vi "SM-SG Main.vi"() -> ()   [LabVIEW 2018]
doc: "Gerador de Sinal estruturado em formato de máquina de estados."
uses:
  Controls/Botao_Senoidal.ctl
  Controls/SM-SG State.ctl
  Controls/SM-SG Data.ctl
  <vilib>/DAQmx/write.llb/DAQmx Write (Analog Wfm 1Chan NSamp).vi
  <vilib>/Waveform/WDTOps.llb/WDT Append Waveforms DBL.vi
  <vilib>/DAQmx/create/channels.llb/DAQmx Create Channel (AO-Voltage-Basic).vi
  <vilib>/DAQmx/configure/timing.llb/DAQmx Timing (Sample Clock).vi
  <vilib>/DAQmx/miscellaneous.llb/DAQmx Fill In Error Info.vi
  <vilib>/measure/NI_MABase.lvlib
  <resource>/objmgr/daqmx.rc
panel:
  in  "% Descida":dbl(knob)=25.01013479174359 max=100.0 step=1.0 scale=0.0..100.0
  in  "% High":dbl(knob)=25.0 min=0.0 max=100.0 step=1.0 scale=0.0..100.0
  in  "% Subida":dbl(knob)=25.0 min=0.0 max=100.0 step=1.0 scale=0.0..100.0
  in  "physical channels 2":tag
  in  "Duty Cycle":dbl(knob) min=0.0 max=100.0 step=1.0 scale=0.0..100.0
  in  "Fase":dbl(knob) min=-180.0 max=180.0 step=5.0 scale=-180.0..180.0
  in  "Offset":dbl(slide) min=-5.5 max=5.5 step=0.1 scale=-5.5..5.5
  in  "Ciclos":i64(knob)=1 min=1 max=10 scale=1.0..10.0
  in  "Frequência":dbl=1.0 min=0.01 max=100000.0 step=0.001
  in  "Amplitude [Vp]":dbl(knob)=5.1000000000000005 caption="Amplitude" min=0.0 max=10.0 step=0.01 scale=0.0..10.0
  in  "Tipo de forma de onda":T2
  in  "Validar":bool
  in  "Parar":bool
  in  "Remove":bool
  out "Xf":dbl
  out "X0":dbl
  in  "Gerar":bool
  out "Sinal":waveform(dbl)(graph)={"t0"=timestamp(0 s since 1904-01-01), "dt"=0.0002, "Y"=[]}
  out "Onda":waveform(dbl)(graph)
  in  "Abrir":bool
  in  "Salvar":bool
  in  "Limpa":bool
  in  "Adicionar":bool
  in  "Stop Button":bool
  # "Onda Configurada"
  # "Configurações da Onda"
  # "Sinal Construído"
  # "Edição do Sinal Construído"
  # "Geração do Sinal"
  # "Cursores"
  # "Canal de Saída"
  # "X1"
  # "X2"
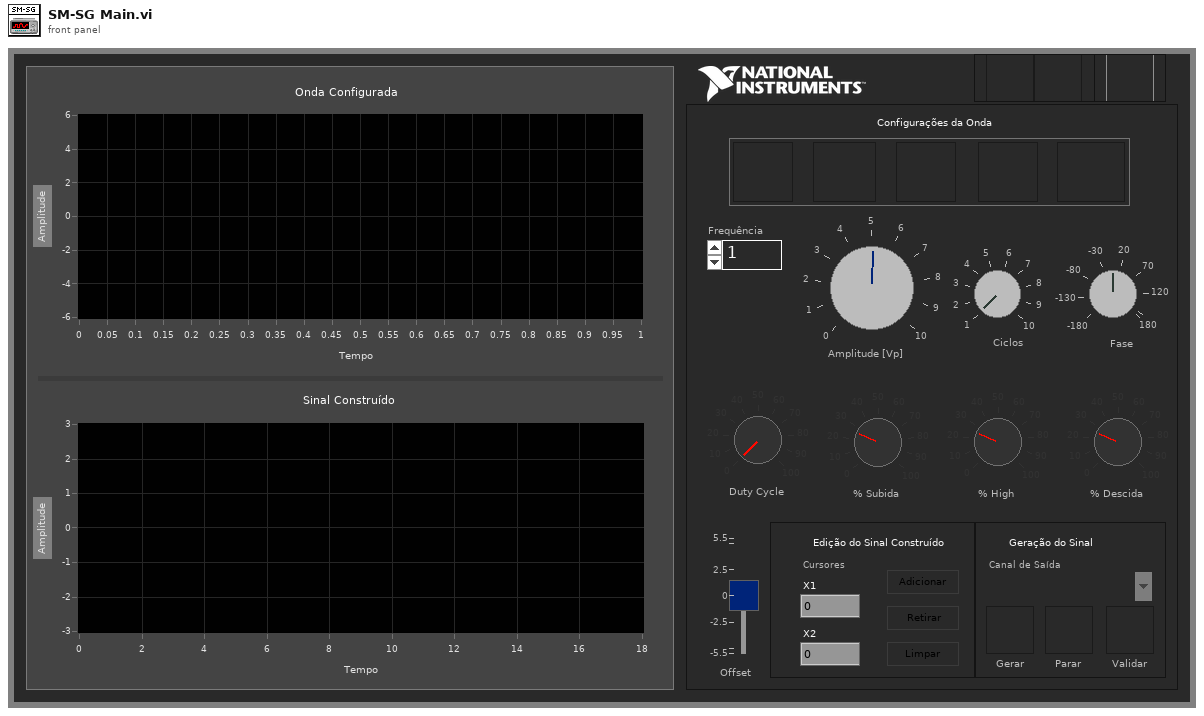
[diagram p1: front panel]
types:
  T1 = typedef "Botao_Senoidal.ctl" = bool
  T2 = cluster{"Sine Wave":T1, "Triangle Wave":bool, "Square Wave":bool, "Sawtooth":bool, "Trapezoidal":bool}
  T3 = typedef "SM-SG Data.ctl" = cluster{"Onda":waveform(dbl), "Sinal":waveform(dbl), "Parâmetros Onda Trapezoidal":cluster{"% Subida ":dbl, "% High ":dbl, "% Descida ":dbl}, "SinalGerado":waveform(dbl), "Analog Output":refnum<k21>, "Analog Input":refnum<k21>, "Tipo de forma de onda ":enum16{"Sine Wave", "Triangle Wave", "Square Wave", "Sawtooth Wave", "Trapezoidal Wave"}, "Amplitude ":dbl, "Frequencia ":dbl, "Ciclos ":dbl, "Fase ":dbl, "Offset":dbl, "Duty Cycle ":dbl}
  T4 = typedef "SM-SG State.ctl" = enum16{"Inicio", "Aguarda Evento", "Desenha Onda", "Mostra Onda", "Mostra Sinal", "Limpa Gráfico", "Adicionar", "Remover", "Salvar", "Carregar", "Gera onda", "Valida onda", "Parar geração", "Gerenciador Erro", "Sair"}
  T5 = enum16{"Sine Wave", "Triangle Wave", "Square Wave", "Sawtooth Wave", "Trapezoidal Wave"}
  T6 = enum16{"open", "open or create", "create or replace", "create", "open (read-only)"}
  T7 = enum16{"Sine Wave", "Triangle Wave", "Square Wave", "Sawtooth Wave", "Trapezoidal Wave"}[]
  T8 = cluster{"% Subida ":dbl, "% High ":dbl, "% Descida ":dbl}
  T9 = typedef "LVCursorListTypeDef.ctl" = cluster{"Name":string, "Color":u32, "Style":u8, "Point Style":u8, "Name Visible":bool, "Allow Drag":bool, "Cursor Mode":u32, "Plot":i32, "Index":i32, "Position":cluster{"X":dbl, "Y":dbl}, "X Scale":u32, "Y Scale":u32, "Watch Plots":i32[], "Watch All Plots":bool, "Plot Area":i32, "Label Offset":cluster{"X":dbl, "Y":dbl}}[]
  T10 = cluster{"CrsrList[0]":cluster{"Name":string, "Color":u32, "Style":u8, "Point Style":u8, "Name Visible":bool, "Allow Drag":bool, "Cursor Mode":u32, "Plot":i32, "Index":i32, "Position":cluster{"X":dbl, "Y":dbl}, "X Scale":u32, "Y Scale":u32, "Watch Plots":i32[], "Watch All Plots":bool, "Plot Area":i32, "Label Offset":cluster{"X":dbl, "Y":dbl}}, "CrsrList[1]":cluster{"Name":string, "Color":u32, "Style":u8, "Point Style":u8, "Name Visible":bool, "Allow Drag":bool, "Cursor Mode":u32, "Plot":i32, "Index":i32, "Position":cluster{"X":dbl, "Y":dbl}, "X Scale":u32, "Y Scale":u32, "Watch Plots":i32[], "Watch All Plots":bool, "Plot Area":i32, "Label Offset":cluster{"X":dbl, "Y":dbl}}, "CrsrList[2]":cluster{"Name":string, "Color":u32, "Style":u8, "Point Style":u8, "Name Visible":bool, "Allow Drag":bool, "Cursor Mode":u32, "Plot":i32, "Index":i32, "Position":cluster{"X":dbl, "Y":dbl}, "X Scale":u32, "Y Scale":u32, "Watch Plots":i32[], "Watch All Plots":bool, "Plot Area":i32, "Label Offset":cluster{"X":dbl, "Y":dbl}}, "CrsrList[3]":cluster{"Name":string, "Color":u32, "Style":u8, "Point Style":u8, "Name Visible":bool, "Allow Drag":bool, "Cursor Mode":u32, "Plot":i32, "Index":i32, "Position":cluster{"X":dbl, "Y":dbl}, "X Scale":u32, "Y Scale":u32, "Watch Plots":i32[], "Watch All Plots":bool, "Plot Area":i32, "Label Offset":cluster{"X":dbl, "Y":dbl}}, "CrsrList[4]":cluster{"Name":string, "Color":u32, "Style":u8, "Point Style":u8, "Name Visible":bool, "Allow Drag":bool, "Cursor Mode":u32, "Plot":i32, "Index":i32, "Position":cluster{"X":dbl, "Y":dbl}, "X Scale":u32, "Y Scale":u32, "Watch Plots":i32[], "Watch All Plots":bool, "Plot Area":i32, "Label Offset":cluster{"X":dbl, "Y":dbl}}, "CrsrList[5]":cluster{"Name":string, "Color":u32, "Style":u8, "Point Style":u8, "Name Visible":bool, "Allow Drag":bool, "Cursor Mode":u32, "Plot":i32, "Index":i32, "Position":cluster{"X":dbl, "Y":dbl}, "X Scale":u32, "Y Scale":u32, "Watch Plots":i32[], "Watch All Plots":bool, "Plot Area":i32, "Label Offset":cluster{"X":dbl, "Y":dbl}}, "CrsrList[6]":cluster{"Name":string, "Color":u32, "Style":u8, "Point Style":u8, "Name Visible":bool, "Allow Drag":bool, "Cursor Mode":u32, "Plot":i32, "Index":i32, "Position":cluster{"X":dbl, "Y":dbl}, "X Scale":u32, "Y Scale":u32, "Watch Plots":i32[], "Watch All Plots":bool, "Plot Area":i32, "Label Offset":cluster{"X":dbl, "Y":dbl}}, "CrsrList[7]":cluster{"Name":string, "Color":u32, "Style":u8, "Point Style":u8, "Name Visible":bool, "Allow Drag":bool, "Cursor Mode":u32, "Plot":i32, "Index":i32, "Position":cluster{"X":dbl, "Y":dbl}, "X Scale":u32, "Y Scale":u32, "Watch Plots":i32[], "Watch All Plots":bool, "Plot Area":i32, "Label Offset":cluster{"X":dbl, "Y":dbl}}, "CrsrList[8]":cluster{"Name":string, "Color":u32, "Style":u8, "Point Style":u8, "Name Visible":bool, "Allow Drag":bool, "Cursor Mode":u32, "Plot":i32, "Index":i32, "Position":cluster{"X":dbl, "Y":dbl}, "X Scale":u32, "Y Scale":u32, "Watch Plots":i32[], "Watch All Plots":bool, "Plot Area":i32, "Label Offset":cluster{"X":dbl, "Y":dbl}}}
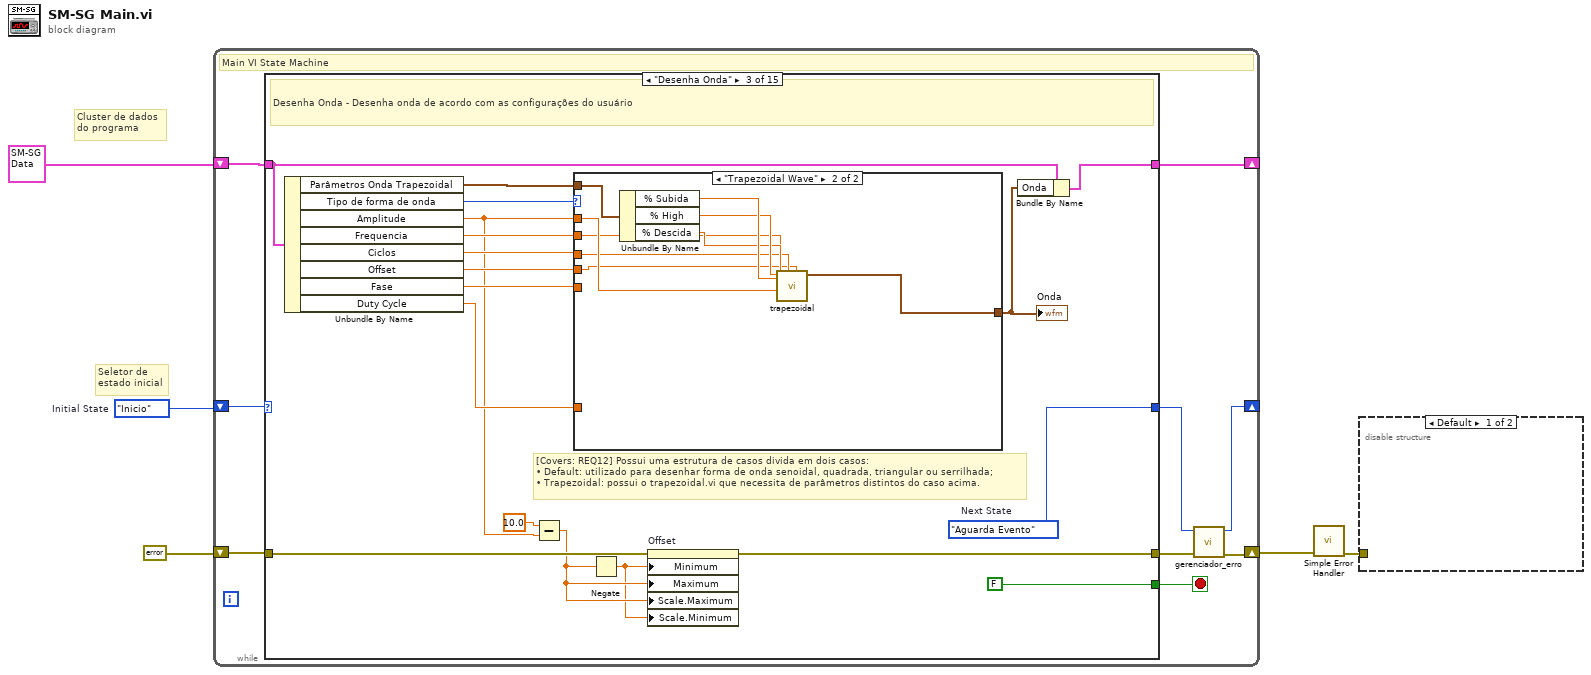
[diagram p0: block diagram]
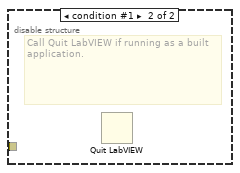
[diagram p2: hidden frame]
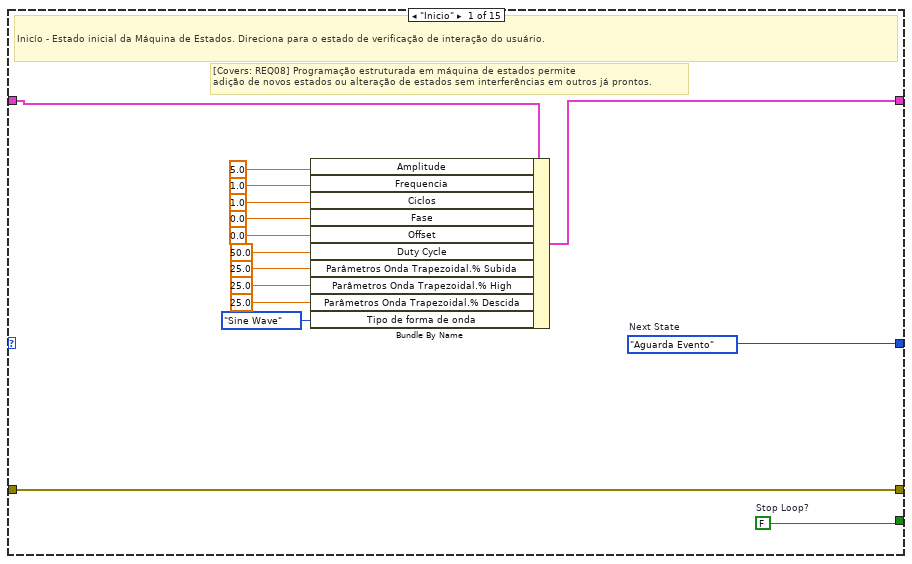
[diagram p3: hidden frame]
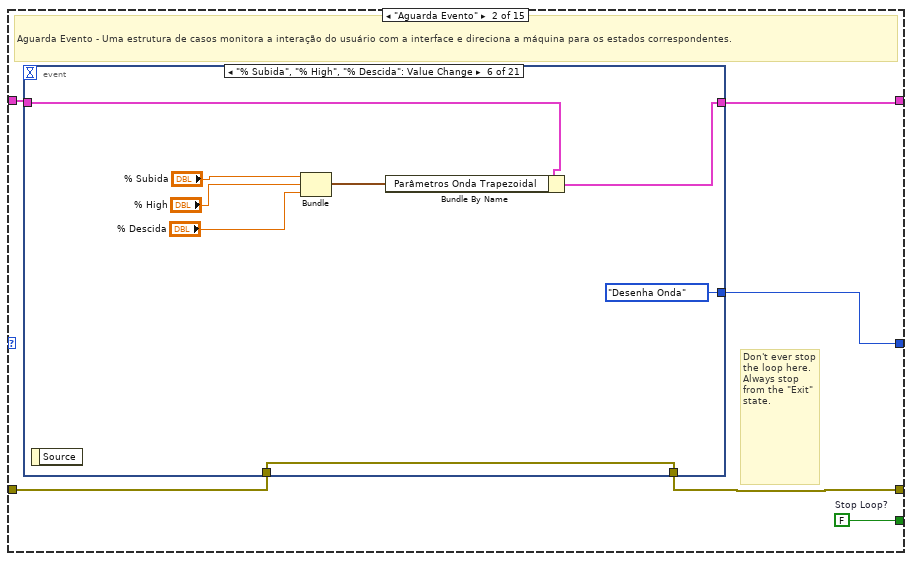
[diagram p4: hidden frame]
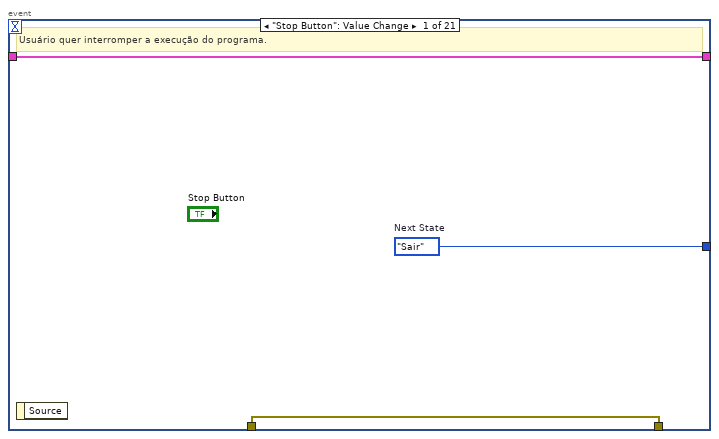
[diagram p5: hidden frame]
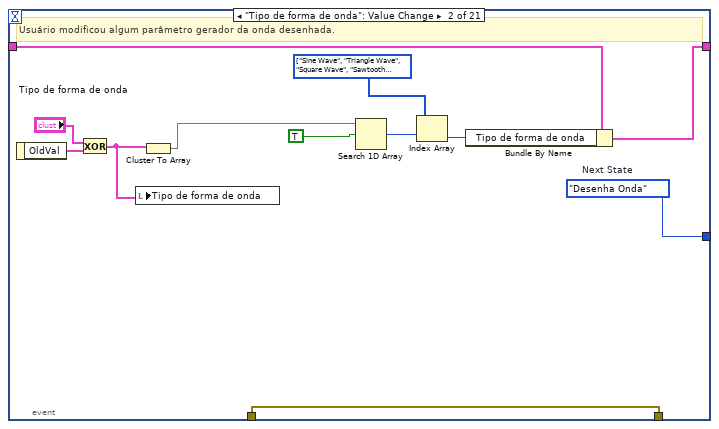
[diagram p6: hidden frame]
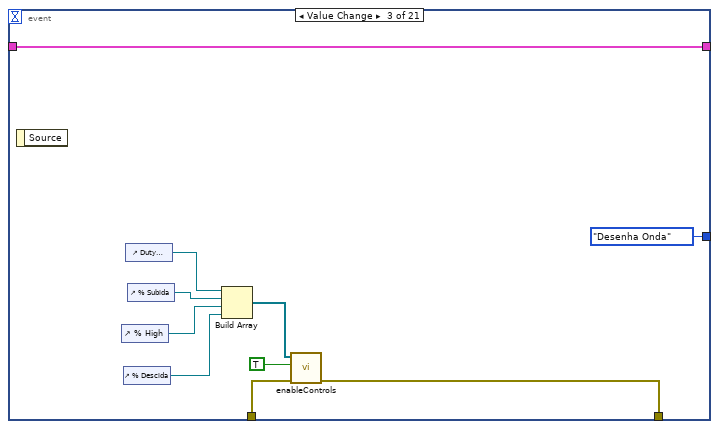
[diagram p7: hidden frame]
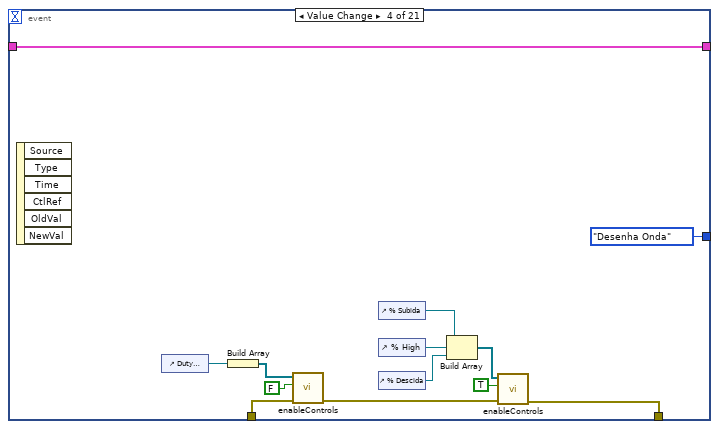
[diagram p8: hidden frame]
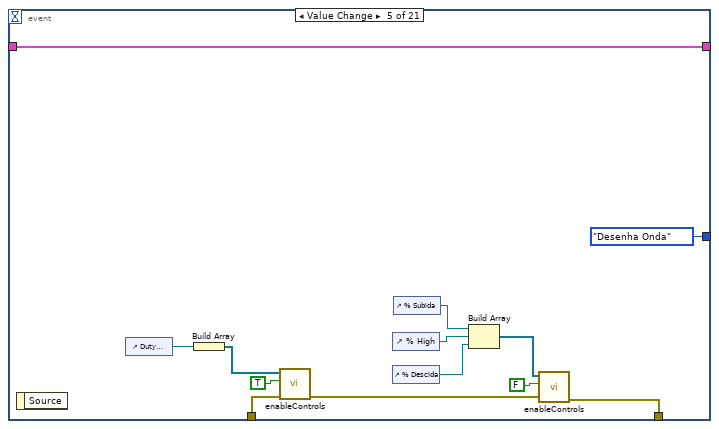
[diagram p9: hidden frame]
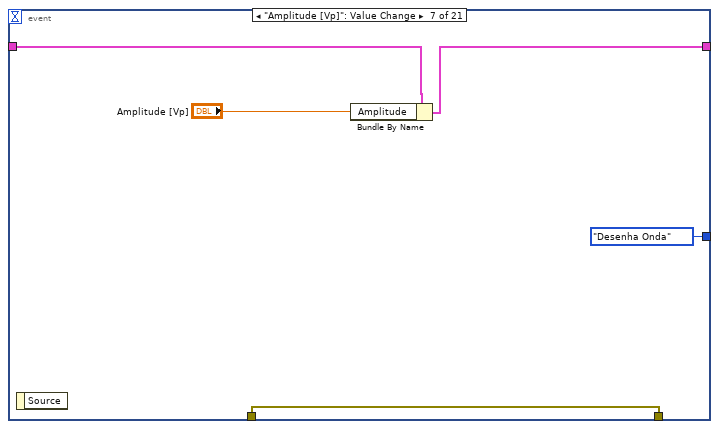
[diagram p10: hidden frame]
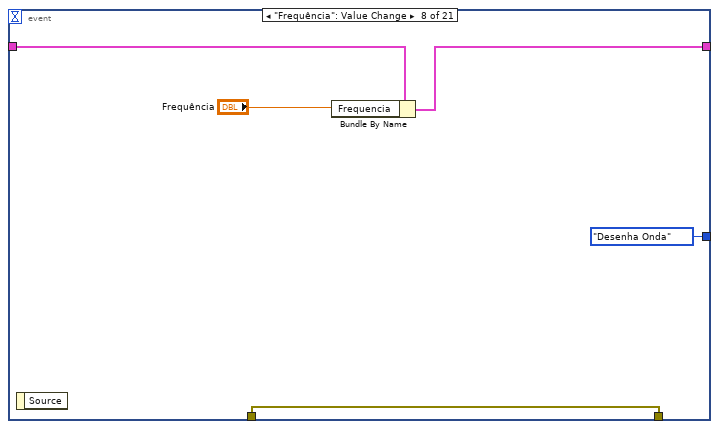
[diagram p11: hidden frame]
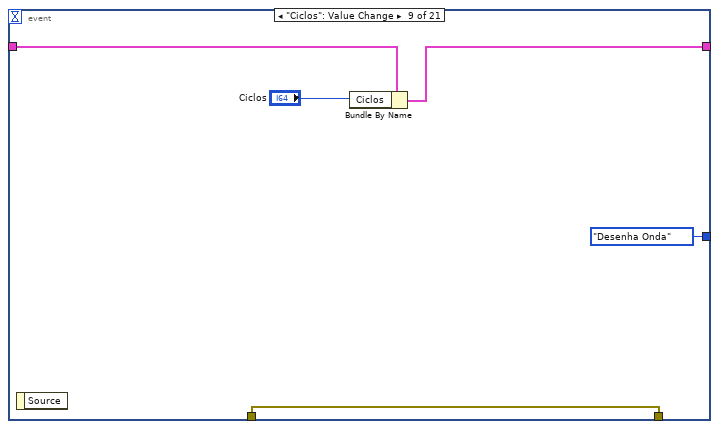
[diagram p12: hidden frame]
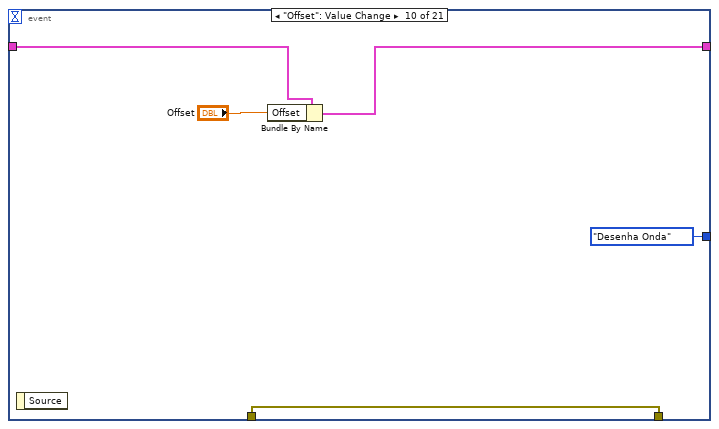
[diagram p13: hidden frame]
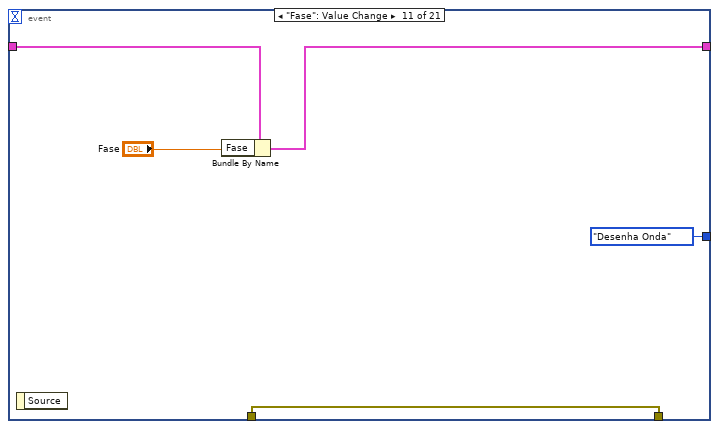
[diagram p14: hidden frame]
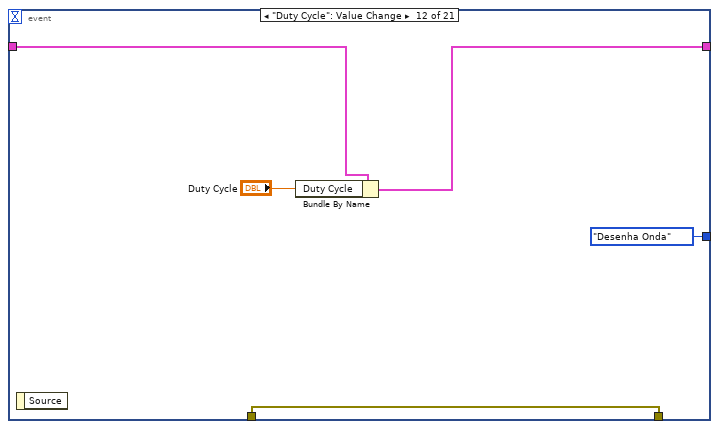
[diagram p15: hidden frame]
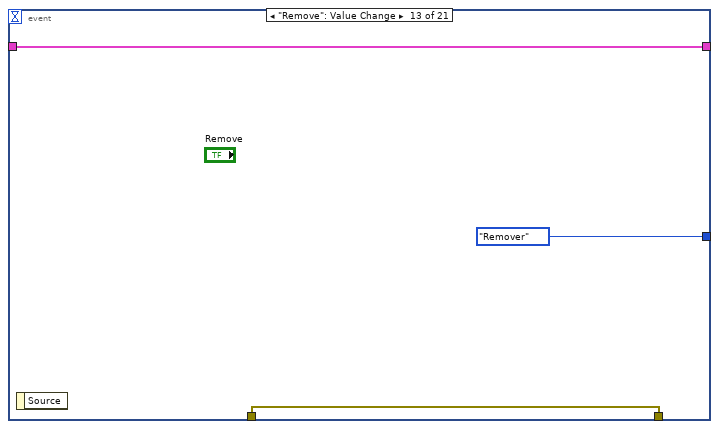
[diagram p16: hidden frame]
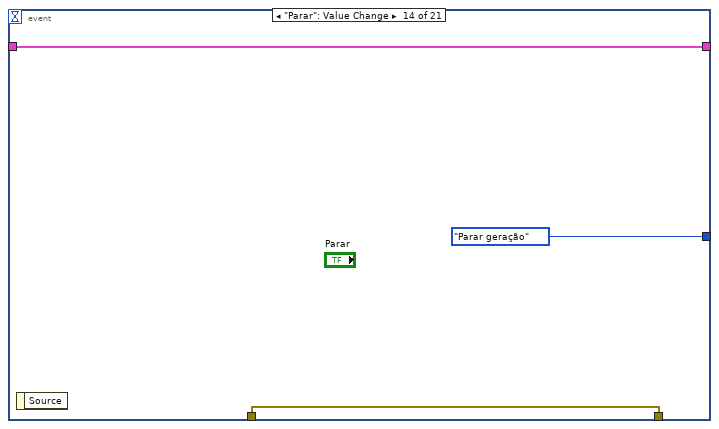
[diagram p17: hidden frame]
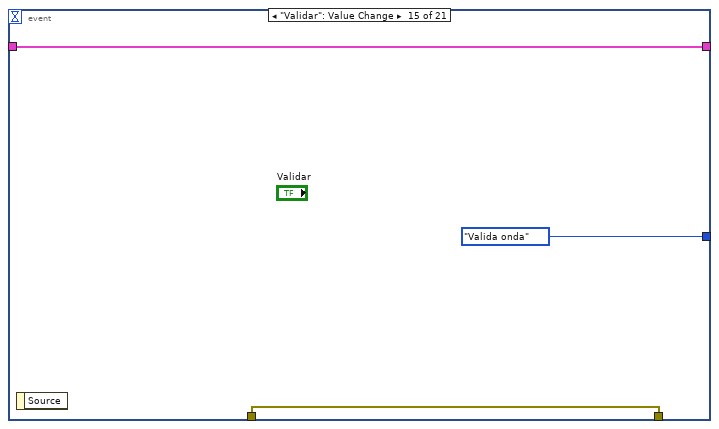
[diagram p18: hidden frame]
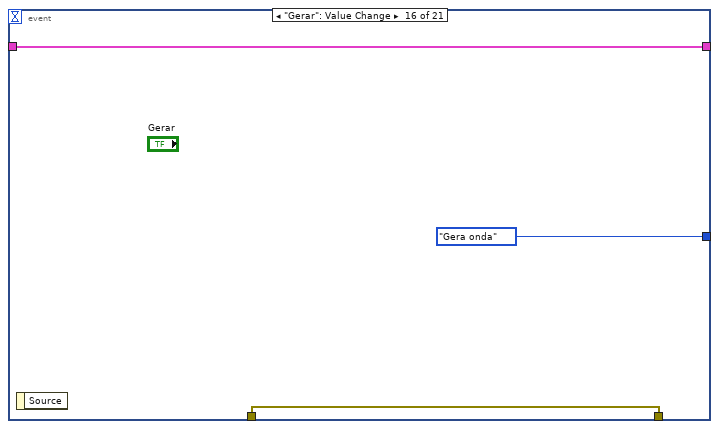
[diagram p19: hidden frame]
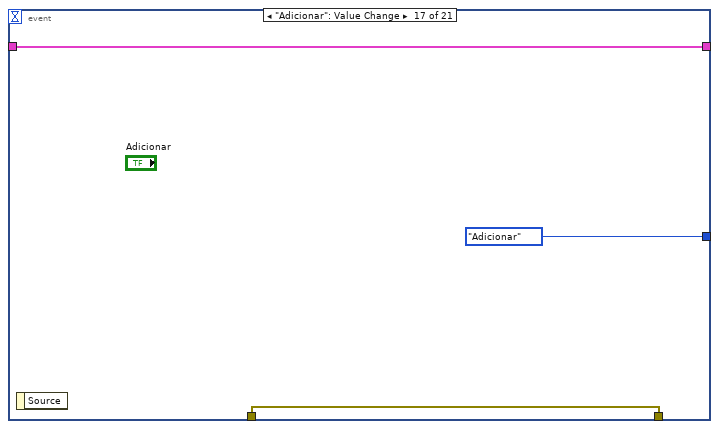
[diagram p20: hidden frame]
diagram:
  w5 = SM-SG_State."Inicio"  # Initial State
  # "Seletor de \nestado inicial"
  # "Cluster de dados\ndo programa"
  n1 = while {
    shift-right: [w7] -> _
    shift-left: w5 -> [w14]
    shift-right: [w11] -> _
    shift-left: T3 {"Onda"={"t0"=timestamp(0 s since 1904-01-01), "dt"=1.0, "Y"=[]}, "Sinal"={"t0"=timestamp(0 s since 1904-01-01), "dt"=1.0, "Y"=[]}, "Parâmetros Onda Trapezoidal"={"% Subida "=0.0, "% High "=0.0, "% Descida "=0.0}, "SinalGerado"={"t0"=timestamp(0 s since 1904-01-01), "dt"=1.0, "Y"=[]}, "Analog Output"="", "Analog Input"="", "Tipo de forma de onda "=enum."Sine Wave", "Amplitude "=0.0, "Frequencia "=0.0, "Ciclos "=1.0, "Fase "=0.0, "Offset"=0.0, "Duty Cycle "=0.0} ("Data") -> [w12]
    shift-right: [w9] -> w3
    shift-left: errorcluster {"status"=FALSE, "code"=0, "source"=""} ("error constant") -> [w13]
    stop <- w6 stop-if-true
    # "Main VI State Machine"
    n2 = case shown="\"Desenha Onda\"" w14 {
      tunnel: [w29 w35 w169 w202 SM-SG_State."Aguarda Evento" SM-SG_State."Mostra Sinal" ("(Value Not Used)") SM-SG_State."Mostra Sinal" ("(Value Not Used)") SM-SG_State."Mostra Sinal" ("(Value Not Used)") SM-SG_State."Aguarda Evento" ("(Value Not Used)") SM-SG_State."Mostra Sinal" ("(Value Not Used)") SM-SG_State."Sair" ("(Value Not Used)") SM-SG_State."Valida onda" ("(Value Not Used)") SM-SG_State."Aguarda Evento" ("(Value Not Used)") SM-SG_State."Aguarda Evento" ("(Value Not Used)") w330] -> w8
      tunnel: [w28 w34 FALSE ("Stop Loop?") FALSE ("Stop Loop?") _ _ _ _ _ _ TRUE ("Stop Loop?") _ _ _ _] -> w6
      tunnel: w12 -> [w26 w33 w165 w191 w203 w219 w223 w230 w256 w285 w289 w303 w321 w326 w331]
      tunnel: [w25 w32 w164 w191 w203 w218 w226 w229 w256 w273 w289 w302 w321 w326 w331] -> w11
      tunnel: [w27 w31 w154 w193 w204 w215 w221 w248 w258 w275 w286 w304 w318 w325 w327] -> w10
      tunnel: w13 -> [w27 w30 w157 _ w205 w215 w222 w248 w253 w269 w286 w315 w319 w323 w328]
      frame "Inicio" {
        w28 = FALSE  # Stop Loop?
        w29 = SM-SG_State."Aguarda Evento"  # Next State
        # "[Covers: REQ08] Programação estruturada em máquina de estados permite \nadição de novos estados ou alteração de estados sem interferências em outros já prontos."
        # "Inicío - Estado inicial da Máquina de Estados. Direciona para o estado de verificação de interação do usuário."
        n3 = Bundle By Name(cluster=w26, "Amplitude"=5.0, "Frequencia"=1.0, "Ciclos"=1.0, "Fase"=0.0, "Offset"=0.0, "Duty Cycle"=50.0, "Parâmetros Onda Trapezoidal.% Subida"=25.0, "Parâmetros Onda Trapezoidal.% High"=25.0, "Parâmetros Onda Trapezoidal.% Descida"=25.0, "Tipo de forma de onda"=T5."Sine Wave") -> (w25:T3)
      }
      frame "Aguarda Evento" {
        w34 = FALSE  # Stop Loop?
        # "Don't ever stop the loop here. Always stop from the \"Exit\" state."
        # "Aguarda Evento - Uma estrutura de casos monitora a interação do usuário com a interface e direciona a máquina para os estados correspondentes."
        n4 = event shown="[5] \"% Subida\", \"% High\", \"% Descida\": Value Change" {
          selector: _ -> [_ _ _ _ _ _ _ _ _ _ _ _ _ _ _ _ _ _ _ _ _]
          dyn-events: _ -> [_ _ _ _ _ _ _ _ _ _ _ _ _ _ _ _ _ _ _ _ _]
          timeout: _ -> [_ _ _ _ _ _ _ _ _ _ _ _ _ _ _ _ _ _ _ _ _]
          tunnel: [w38 w50 SM-SG_State."Desenha Onda" ("Next State") SM-SG_State."Desenha Onda" ("Next State") SM-SG_State."Desenha Onda" ("Next State") SM-SG_State."Desenha Onda" ("Next State") SM-SG_State."Desenha Onda" ("Next State") SM-SG_State."Desenha Onda" ("Next State") SM-SG_State."Desenha Onda" ("Next State") SM-SG_State."Desenha Onda" ("Next State") SM-SG_State."Desenha Onda" ("Next State") SM-SG_State."Desenha Onda" ("Next State") SM-SG_State."Remover" ("Next State") SM-SG_State."Parar geração" ("Next State") SM-SG_State."Valida onda" ("Next State") SM-SG_State."Gera onda" ("Next State") SM-SG_State."Adicionar" ("Next State") SM-SG_State."Mostra Sinal" ("Next State") SM-SG_State."Limpa Gráfico" ("Next State") SM-SG_State."Carregar" ("Next State") SM-SG_State."Salvar" ("Next State")] -> w35
          tunnel: w33 -> [w37 w46 w60 w73 w74 w88 w98 w102 w107 w113 w118 w123 w126 w129 w132 w135 w138 w141 w144 w147 w150]
          tunnel: [w37 w45 w60 w73 w74 w87 w96 w101 w106 w112 w117 w122 w126 w129 w132 w135 w138 w141 w144 w147 w150] -> w32
          tunnel: w30 -> [w36 w42 w59 w71 w85 w94 w95 w100 w105 w110 w115 w120 w125 w128 w131 w134 w137 w140 w143 w146 w149]
          tunnel: [w36 w42 w52 w66 w83 w94 w95 w100 w105 w110 w115 w120 w125 w128 w131 w134 w137 w140 w143 w146 w149] -> w31
          event "Stop Button": Value Change {
            w38 = SM-SG_State."Sair"  # Next State
            # "Usuário quer interromper a execução do programa."
            n5 = event-data() -> ()  [unwired: 1 in, 1 out]
          }
          event "Tipo de forma de onda": Value Change {
            w48 = T7 [enum."Sine Wave", enum."Triangle Wave", enum."Square Wave", enum."Sawtooth Wave", enum."Trapezoidal Wave"] items=["Sine Wave", "Triangle Wave", "Square Wave", "Sawtooth Wave", "Trapezoidal Wave"] ("array")
            w50 = SM-SG_State."Desenha Onda"  # Next State
            # "Usuário modificou algum parâmetro gerador da onda desenhada."
            n6 = event-data() -> ("OldVal"=w43:T2)  [unwired: 1 in]
            n7 = Exclusive Or(1:w43, 2:"Tipo de forma de onda") -> (0:w41:T2)
            n8 = local write "Tipo de forma de onda"(w41) -> ()
            n9 = Cluster To Array(cluster=w41) -> (array=w40:T1[])
            n10 = Search 1D Array(1D array=w40, element=TRUE) -> (index of element=w49:i32)  [unwired: 1 in]
            n11 = Index Array(array=w48, index=w49) -> (element=w47:T5)
            n12 = Bundle By Name(cluster=w46, "Tipo de forma de onda"=w47) -> (w45:T3)
          }
          event "Tipo de forma de onda.Triangle Wave", "Tipo de forma de onda.Sawtooth": Value Change {
            n13 = event-data() -> ()  [unwired: 1 in, 1 out]
            n14 = control-ref of="% High"() -> (w55:refnum<vi>)
            n15 = control-ref of="% Descida"() -> (w54:refnum<vi>)
            n16 = control-ref of="Duty Cycle"() -> (w58:refnum<vi>)
            n17 = control-ref of="% Subida"() -> (w56:refnum<vi>)
            n18 = Build Array(w58, w56, w55, w54) -> (w53:refnum<vi>[])
            n19 = call "enableControls.vi"("Error In"=w59, "Disable?"=TRUE, "Controls"=w53) -> ("Error Out"=w52:errorcluster)  [unwired: 8 in]
          }
          event "Tipo de forma de onda.Square Wave": Value Change {
            n20 = event-data() -> ()  [unwired: 1 in, 6 out]
            n21 = control-ref of="Duty Cycle"() -> (w70:refnum<vi>)
            n22 = Build Array(w70) -> (w69:refnum<vi>[])
            n23 = call "enableControls.vi"("Error In"=w71, "Disable?"=FALSE, "Controls"=w69) -> ("Error Out"=w67:errorcluster)  [unwired: 8 in]
            n24 = control-ref of="% Subida"() -> (w65:refnum<vi>)
            n25 = control-ref of="% High"() -> (w64:refnum<vi>)
            n26 = control-ref of="% Descida"() -> (w63:refnum<vi>)
            n27 = Build Array(w65, w64, w63) -> (w62:refnum<vi>[])
            n28 = call "enableControls.vi"("Error In"=w67, "Disable?"=TRUE, "Controls"=w62) -> ("Error Out"=w66:errorcluster)  [unwired: 8 in]
          }
          event "Tipo de forma de onda.Trapezoidal": Value Change {
            n29 = event-data() -> ()  [unwired: 1 in, 1 out]
            n30 = control-ref of="Duty Cycle"() -> (w82:refnum<vi>)
            n31 = Build Array(w82) -> (w81:refnum<vi>[])
            n32 = call "enableControls.vi"("Error In"=w85, "Disable?"=TRUE, "Controls"=w81) -> ("Error Out"=w84:errorcluster)  [unwired: 8 in]
            n33 = control-ref of="% High"() -> (w77:refnum<vi>)
            n34 = control-ref of="% Descida"() -> (w76:refnum<vi>)
            n35 = control-ref of="% Subida"() -> (w78:refnum<vi>)
            n36 = Build Array(w78, w77, w76) -> (w75:refnum<vi>[])
            n37 = call "enableControls.vi"("Error In"=w84, "Disable?"=FALSE, "Controls"=w75) -> ("Error Out"=w83:errorcluster)  [unwired: 8 in]
          }
          event "% Subida", "% High", "% Descida": Value Change {
            n38 = event-data() -> ()  [unwired: 1 in, 1 out]
            n39 = Bundle("% Subida"="% Subida", "% High"="% High", "% Descida"="% Descida") -> (w89:T8)  [unwired: 1 in]
            n40 = Bundle By Name(cluster=w88, "Parâmetros Onda Trapezoidal"=w89) -> (w87:T3)
          }
          event "Amplitude [Vp]": Value Change {
            n41 = event-data() -> ()  [unwired: 1 in, 1 out]
            n42 = Bundle By Name(cluster=w98, "Amplitude"="Amplitude [Vp]") -> (w96:T3)
          }
          event "Frequência": Value Change {
            n43 = event-data() -> ()  [unwired: 1 in, 1 out]
            n44 = Bundle By Name(cluster=w102, "Frequencia"="Frequência") -> (w101:T3)
          }
          event "Ciclos": Value Change {
            n45 = event-data() -> ()  [unwired: 1 in, 1 out]
            n46 = Bundle By Name(cluster=w107, "Ciclos"="Ciclos") -> (w106:T3)
          }
          event "Offset": Value Change {
            n47 = event-data() -> ()  [unwired: 1 in, 1 out]
            n48 = Bundle By Name(cluster=w113, "Offset"="Offset") -> (w112:T3)
          }
          event "Fase": Value Change {
            n49 = event-data() -> ()  [unwired: 1 in, 1 out]
            n50 = Bundle By Name(cluster=w118, "Fase"="Fase") -> (w117:T3)
          }
          event "Duty Cycle": Value Change {
            n51 = event-data() -> ()  [unwired: 1 in, 1 out]
            n52 = Bundle By Name(cluster=w123, "Duty Cycle"="Duty Cycle") -> (w122:T3)
          }
          event "Remove": Value Change {
            n53 = event-data() -> ()  [unwired: 1 in, 1 out]
          }
          event "Parar": Value Change {
            n54 = event-data() -> ()  [unwired: 1 in, 1 out]
          }
          event "Validar": Value Change {
            n55 = event-data() -> ()  [unwired: 1 in, 1 out]
          }
          event "Gerar": Value Change {
            n56 = event-data() -> ()  [unwired: 1 in, 1 out]
          }
          event "Adicionar": Value Change {
            n57 = event-data() -> ()  [unwired: 1 in, 1 out]
          }
          event "Sinal": Cursor Move {
            n58 = event-data() -> ()  [unwired: 1 in, 1 out]
          }
          event "Limpa": Value Change {
            n59 = event-data() -> ()  [unwired: 1 in, 1 out]
          }
          event "Abrir": Value Change {
            n60 = event-data() -> ()  [unwired: 1 in, 1 out]
          }
          event "Salvar": Value Change {
            # "Usuário quer salvar a forma de onda desenhada."
            n61 = event-data() -> ()  [unwired: 1 in, 1 out]
          }
        }
      }
      frame "Desenha Onda" {
        w169 = SM-SG_State."Aguarda Evento"  # Next State
        # "[Covers: REQ12] Possui uma estrutura de casos divida em dois casos:\n• Default: utilizado para desenhar forma de onda senoidal, quadrada, triangular ou serrilhada;\n• Trapezoidal: possui o trapezoidal.vi que necessita de parâmetros distintos do caso acima."
        # "Desenha Onda - Desenha onda de acordo com as configurações do usuário"
        n62 = Unbundle By Name(w165) -> ("Parâmetros Onda Trapezoidal"=w167:T8, "Tipo de forma de onda"=w163:T5, "Amplitude"=w155:dbl, "Frequencia"=w162:dbl, "Ciclos"=w161:dbl, "Offset"=w160:dbl, "Fase"=w158:dbl, "Duty Cycle"=w159:dbl)
        n63 = Subtract(x=10.0, y=w155) -> (x-y=w153:dbl)
        n64 = case shown="\"Trapezoidal Wave\"" w163 {
          selector: w163 -> [w176 _]
          tunnel: [w181 w189] -> w166
          tunnel: w167 -> [_ w190]
          tunnel: w155 -> [w173 w185]
          tunnel: w162 -> [w174 w184]
          tunnel: w161 -> [w171 w183]
          tunnel: w160 -> [w175 w182]
          tunnel: w159 -> [w172 _]
          tunnel: w158 -> [w170 _]
          frame "Sine Wave", Default {
            w177 = 1000000.0
            n65 = Divide(x=w177, y=w174) -> (x/y=w178:dbl)
            n66 = Multiply(x=w178, y=w171) -> (x*y=w179:dbl)
            n67 = Bundle(w177, w179) -> (w180:cluster{dbl, dbl})  [unwired: 1 in]
            n68 = call <vilib>:"Basic Function Generator.vi"("offset"=w175, "square wave duty cycle (%)"=w172, "sampling info"=w180, "signal type"=w176, "phase"=w170, "amplitude"=w173, "frequency"=w174) -> ("signal out"=w181:waveform(dbl))  [unwired: 2 in, 2 out]
          }
          frame "Trapezoidal Wave" {
            n69 = Unbundle By Name(w190) -> ("% Subida"=w188:dbl, "% High"=w187:dbl, "% Descida"=w186:dbl)
            n70 = call "trapezoidal.vi"("Offset"=w182, "Ciclos"=w183, "%Subida"=w188, "Frequencia"=w184, "Amplitude"=w185, "%Descida"=w186, "%Alto"=w187) -> ("Waveform Graph"=w189:waveform(dbl))  [unwired: 4 in]
          }
        }
        "Onda" <- w166
        n71 = Negate(x=w153) -> (-x=w152:dbl)
        n72 = property on="Offset" class="Slide (strict)"(error in=w157, "Minimum"=w152, "Maximum"=w153, "Scale.Maximum"=w153, "Scale.Minimum"=w152) -> (error out=w154:errorcluster)  [unwired: 1 in, 1 out]
        n73 = Bundle By Name(cluster=w165, "Onda"=w166) -> (w164:T3)
      }
      frame "Mostra Onda" {
        w202 = SM-SG_State."Aguarda Evento"  # Next State
        # "Estado vazio"
        n74 = Unbundle By Name(w191) -> ("Frequencia"=w199:dbl, "Ciclos"=w197:dbl, "Amplitude"=w195:dbl)
        n75 = Reciprocal(x=w199) -> (1/x=w198:dbl)
        n76 = Multiply(x=w198, y=w197) -> (x*y=w192:dbl)
        n77 = property on="Onda" class="WFGraph (strict)"("XScale.Maximum"=w192, "XScale.Minimum"=0.0 ("X Scale.Range:Minimum")) -> (error out=w194:errorcluster)  [unwired: 2 in, 1 out]
        n78 = Negate(x=w195) -> (-x=w196:dbl)
        n79 = property on="Onda" class="WFGraph (strict)"(error in=w194, "YScale.Minimum"=w196, "YScale.Maximum"=w195) -> (error out=w193:errorcluster)  [unwired: 1 in, 1 out]
      }
      frame "Mostra Sinal" {
        # "Mostra Sinal - Exibe o sinal total desejado e construido pelo usuário pelos estados de adição e remoção."
        n80 = property on="Sinal" class="WFGraph (strict)"(error in=w205) -> (error out=w204:errorcluster, "CrsrList"=w209:T9)  [unwired: 1 in, 1 out]
        n81 = Array To Cluster(array=w209) -> (cluster=w208:T10)
        n82 = Unbundle By Name(w208) -> ("CrsrList[0].Position.X"=→"X0":dbl, "CrsrList[1].Position.X"=→"Xf":dbl)
        n83 = Unbundle By Name(w203) -> ("Sinal"=w210:waveform(dbl))
        n84 = Reciprocal(x=1000000.0) -> (1/x=w212:dbl)
        n85 = Bundle By Name(cluster=w210, "dt"=w212) -> (→"Sinal":waveform(dbl))
      }
      frame "Limpa Gráfico" {
        # "Limpa Gráfico - Limpa o gráfico de sinal desenhado"
        n86 = Bundle By Name(cluster=w219, "Sinal"=waveform(dbl) {"t0"=timestamp(0 s since 1904-01-01), "dt"=1.0, "Y"=[]} ("Waveform")) -> (w218:T3)
      }
      frame "Adicionar" {
        # "Adicionar - Adiciona ao sinal a forma de onda atual configurada pelo usuário. [Covers: REQ13]"
        n87 = Unbundle By Name(w223) -> ("Sinal"=w228:waveform(dbl), "Onda"=w227:waveform(dbl))
        n88 = call-poly <vilib>:"Append Waveforms.vi"("waveform B"=w227, "waveform A"=w228) -> ("waveform out"=w225:waveform(dbl))  [unwired: 8 in, 1 out]
        n89 = property on="Sinal" class="WFGraph (strict)"(error in=w222, "Cursor.Cursor X"=0.5 ("Cursor.Cursor Position:Cursor X")) -> (error out=w221:errorcluster)  [unwired: 1 in, 1 out]
        n90 = Bundle By Name(cluster=w223, "Sinal"=w225) -> (w226:T3)
      }
      frame "Remover" {
        w244 = 1000000.0
        # "calcula o número de amostras\nequivalente ao intervalo a ser eliminado"
        # "verifica qual cursor possui o menor valor de x\ne relaciona-os corretamente para prosseguir com a lógica"
        # "tf"
        # "t0"
        # "Remover - Remove do sinal a forma de onda selecionada entre os cursores pelo usuário. [Covers: REQ13]"
        n91 = local read "X0"() -> (w246:dbl)
        n92 = local read "Xf"() -> (w247:dbl)
        n93 = Less?(x=w246, y=w247) -> (x < y?=w231:bool)
        n94 = Unbundle By Name(w230) -> ("Sinal"=w243:waveform(dbl))
        n95 = case shown="False" w231 {
          tunnel: w247 -> [w249 w251]
          tunnel: w246 -> [w250 w252]
          tunnel: [w249 w252] -> w245
          tunnel: [w250 w251] -> w236
          frame False {
          }
          frame True {
          }
        }
        n96 = Multiply(x=w244, y=w245) -> (x*y=w232:dbl)
        n97 = Multiply(x=w244, y=w236) -> (x*y=w238:dbl)
        n98 = To Long Integer(number=w232) -> (32bit integer=w234:i32)
        n99 = To Long Integer(number=w238) -> (32bit integer=w235:i32)
        n100 = Unbundle By Name(w243) -> ("dt"=w241:dbl, "Y"=w237:dbl[])
        n101 = Subtract(x=w235, y=w234) -> (x-y=w233:i32)
        n102 = Delete From Array(array=w237, length=w233, index=w234) -> (array with subset deleted=w242:dbl[])  [unwired: 1 out]
        n103 = Bundle By Name("dt"=w241, "Y"=w242) -> (w240:waveform(dbl))  [unwired: 1 in]
        n104 = Bundle By Name(cluster=w230, "Sinal"=w240) -> (w229:T3)
      }
      frame "Salvar" {
        # "#Melhorar Documentar propriedades do TDMS"
        # "Salvar - Salva em TDMS o sinal fianl gerado pelo usuário. [Covers: REQ14]"
        n105 = Default Directory() -> (w254:path)
        n106 = call "File Dialog"("start path"=w254, "default name"="wave_", "error in"=w253) -> ("selected path"=w264:path, "error out"=w265:errorcluster)  [unwired: 9 in, 2 out]
        n107 = TDMS Open(5:TRUE ("create index file? (T)"), 8:w265, 10:T6."create or replace" ("operation (0:open)"), 11:w264) -> (0:w260:errorcluster, 3:w261:refnum<k34>)  [unwired: 3 in]
        n108 = Unbundle By Name(w256) -> ("Sinal"=w255:waveform(dbl))
        n109 = TDMS Write(0:w261, 1:enum16{"decimated", "interleaved"}."decimated" ("data layout (0:decimated)"), 9:w255, 11:w260) -> (4:w268:refnum<k34>, 15:w259:errorcluster)  [unwired: 2 in, 2 out]
        n110 = TDMS Close(8:w259, 11:w268) -> (0:w258:errorcluster)  [unwired: 1 out]
      }
      frame "Carregar" {
        # "Carregar - Carrega uma arquivo TDMS com forma de onda salva anteriormente para o gráfico 'Sinal'. [Covers: REQ14]"
        n111 = Default Directory() -> (w270:path)
        n112 = call "File Dialog2"("start path"=w270, "prompt"="Encontre o arquivo que \ndeseja carregar", "error in"=w269, "pattern (all files)"="*.tdms") -> ("selected path"=w279:path, "error out"=w278:errorcluster)  [unwired: 8 in, 2 out]
        n113 = TDMS Open(8:w278, 10:T6."open" ("operation (0:open)"), 11:w279) -> (0:w281:errorcluster, 3:w282:refnum<k34>)  [unwired: 4 in]
        n114 = TDMS Read(0:w282, 11:w281, 12:waveform(dbl) {"t0"=timestamp(0 s since 1904-01-01), "dt"=1.0, "Y"=[]} ("Waveform")) -> (4:w284:refnum<k34>, 10:w272:waveform(dbl), 15:w283:errorcluster)  [unwired: 5 in, 3 out]
        n115 = Bundle By Name(cluster=w285, "Sinal"=w272) -> (w273:T3)
        n116 = TDMS Close(8:w283, 11:w284) -> (0:w275:errorcluster)  [unwired: 1 out]
      }
      frame "Sair" {
        # "Sair - Para a execução do programa."
      }
      frame "Gera onda" {
        w295 = 10097 items=["Allow Regeneration"=10097, "Do Not Allow Regeneration"=10158] ("RegenMode")
        w299 = 10123 items=["Finite Samples"=10178, "Continuous Samples"=10123, "Hardware Timed Single Point"=12522] ("sample mode")
        w309 = 10083 items=["Default"=-1, "RSE"=10083, "Differential"=10106, "Pseudodifferential"=12529] ("output terminal configuration")
        w312 = 10348 items=["Volts"=10348, "From Custom Scale"=10065] ("units")
        # "Frequência de Geração.\n[Covers: REQ17]"
        # "canal de saída"
        # "Valor max e min de tensão\n[Covers: REQ16]"
        # "unidade"
        # "nome do canal"
        # "Gera Onda - Gera uma onda no hardware a partir do sinal gerado pelo usuário. [Covers: REQ15]"
        n117 = call <vilib>:"DAQmx Create Task.vi"("auto cleanup"=TRUE, "error in"=w315) -> ("task out"=w293:refnum<k21>, "error out"=w314:errorcluster)  [unwired: 12 in]
        n118 = Unbundle By Name(w303) -> ("Sinal"=w300:waveform(dbl))
        n119 = call-poly <vilib>:"DAQmx Create Virtual Channel.vi"("task in"=w293, "maximum value"=10.0, "minimum value"=-10.0, "output terminal configuration"=w309, "physical channels"="physical channels 2", "name to assign"="Sinal Gerado", "units"=w312, "error in"=w314) -> ("task out"=w297:refnum<k21>, "error out"=w291:errorcluster)  [unwired: 6 in]
        n120 = property class="DAQmx Write"(reference=w297, error in=w291, "RegenMode"=w295) -> (reference out=w296:refnum<k21>, error out=w298:errorcluster)
        n121 = call-poly <vilib>:"DAQmx Timing.vi"("task/channels in"=w296, "sample mode"=w299, "rate"=1000000.0, "source"=tag "", "error in"=w298) -> ("task out"=w306:refnum<k21>, "error out"=w305:errorcluster)  [unwired: 9 in]
        n122 = call-poly <vilib>:"DAQmx Write.vi"("task/channels in"=w306, "data"=w300, "error in"=w305) -> ("task out"=w308:refnum<k21>, "error out"=w307:errorcluster)  [unwired: 10 in, 1 out]
        n123 = call <vilib>:"DAQmx Start Task.vi"("task/channels in"=w308, "error in"=w307) -> ("task out"=w301:refnum<k21>, "error out"=w304:errorcluster)  [unwired: 12 in]
        n124 = Bundle By Name(cluster=w303, "Analog Output"=w301) -> (w302:T3)
      }
      frame "Valida onda" {
        # "SubVI Launch"
        # "Valida onda - Lança janela de aquisição para visualização da onda gerada pelo NI USB-6251. [Covers: REQ15]"
        n125 = call "Launch VI.vi"("Error In"=w319) -> ("Error Out"=w318:errorcluster)  [unwired: 10 in]
      }
      frame "Parar geração" {
        n126 = Unbundle By Name(w326) -> ("Analog Output"=w322:refnum<k21>)
        n127 = call <vilib>:"DAQmx Clear Task.vi"("task in"=w322, "error in"=w323) -> ("error out"=w325:errorcluster)  [unwired: 13 in]
      }
      frame "Gerenciador Erro" {
        n128 = Unbundle By Name(w328) -> ("code"=w329:i32)  [unwired: 2 out]
        n129 = case shown="43" w329 {
          selector: w329 -> [_ w340 _]
          tunnel: [SM-SG_State."Aguarda Evento" ("(Value Not Used)") w342 SM-SG_State."Aguarda Evento" ("(Value Not Used)")] -> w330
          tunnel: [w332 w334 w349] -> w327
          tunnel: w328 -> [w332 w341 w350]
          frame 0, Default {
          }
          frame -200099 {
            # "F:"
            # "T:"
            # "Erro: Usuário não inseriu o canal de saída para geração do sinal"
            n130 = call <vilib>:"Clear Errors.vi"("error in (no error)"=w341, "specific error code to clear (0: all)"=w340) -> ("error out"=w335:errorcluster)  [unwired: 4 in, 1 out]
            n131 = Two Button Dialog(message="Canal de saída não especificado.", 1:"Cancelar geração" ("F button name (\"Cancel\")"), 2:"Indicar canal" ("T button name (\"OK\")")) -> (T button?=w336:bool)
            n132 = case shown="True" w336 {
              tunnel: [SM-SG_State."Aguarda Evento" ("(Value Not Used)") SM-SG_State."Aguarda Evento" ("(Value Not Used)")] -> w342
              tunnel: w335 -> [w344 w346]
              tunnel: [w344 w345] -> w334
              frame False {
              }
              frame True {
                n133 = invoke on="physical channels 2" class="DAQmxName" method="ObjHighlight"(error in=w346) -> (error out=w345:errorcluster)  [unwired: 2 in, 2 out]
              }
            }
          }
          frame 43 {
            n134 = call <vilib>:"Clear Errors.vi"("error in (no error)"=w350) -> ("error out"=w349:errorcluster)  [unwired: 5 in, 1 out]
          }
        }
      }
    }
    n135 = call "gerenciador_erro.vi"("error in"=w10, "Estado in"=w8) -> ("error out"=w9:errorcluster, "States"=w7:T4)  [unwired: 8 in]
  }
  n136 = call <vilib>:"Simple Error Handler.vi"("error in (no error)"=w3) -> ("error out"=w2:errorcluster)  [unwired: 4 in, 4 out]
  n137 = disable-structure shown="Default" {
    disable-tunnel: w2 -> [_ _]
    frame condition #0 (active) {
    }
    frame condition #1 {
      # "Call Quit LabVIEW if running as a built application."
      n138 = Quit LabVIEW() -> ()  [unwired: 1 in]
    }
  }
